vi "WPI_Camera Registry.vi"(8 "error in (no error)":errorcluster, 9 "Disallow Simulation":bool, 10 "Camera Address":string="192.168.0.90", 11 "Action":T2) -> (0 "error out":errorcluster, 3 "CameraDevRef":T1)   [LabVIEW 2017]
doc: "This software is licensed. Open the labview\\readme\\WPI Robotics Library Open Source License.txt file for more information."
uses:
  <vilib>/Rock Robotics/WPI/Camera/WPI_CameraRegistryActions.ctl
  <vilib>/Rock Robotics/WPI/Camera/WPI_CameraDevRef.ctl
  <vilib>/Rock Robotics/WPI/Camera/WPI_CameraSettings Operations.ctl
  <vilib>/Rock Robotics/WPI/Camera/WPI_CameraSettings Control.ctl
  <vilib>/Rock Robotics/WPI/Camera/WPI_CameraImageSize.ctl
  <vilib>/Rock Robotics/WPI/Camera/WPI_CameraWhite Balance Values.ctl
  <vilib>/Rock Robotics/WPI/Camera/WPI_CameraExposure Values.ctl
  <vilib>/Rock Robotics/WPI/Camera/WPI_CameraExposure Priority Values.ctl
  <vilib>/vision/driver/NI_Vision_Acquisition_Software.lvlib
panel:
  out "Camera Addresses":string[](array[string])
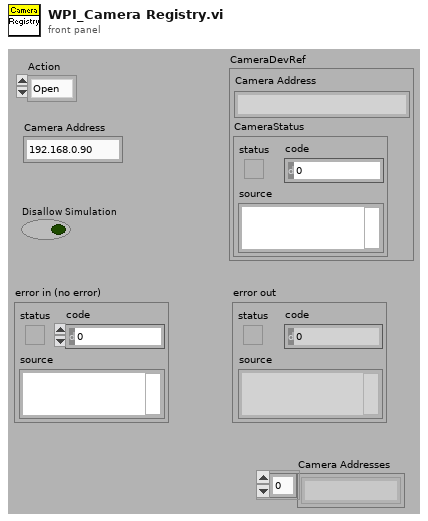
[diagram p1: front panel]
types:
  T1 = typedef "WPI_CameraDevRef.ctl" = cluster{"Camera Address":string, "CameraStatus":errorcluster}
  T2 = typedef "WPI_CameraRegistryActions.ctl" = enum16{"Open", "Close"}
  T3 = typedef "WPI_CameraSettings Control.ctl" = cluster{"FPS":i32, "Compression":i32, "Size":i32, "White Balance":i32, "Brightness":i32, "Sharpness":i32, "Exposure":i32, "Color Level":i32, "Exposure Priority":i32, "Color Enable":i32, "JPG Loop":i32, "MJPG Loop":i32, "Exposure Value":i32}
  T4 = typedef "WPI_CameraSettings Operations.ctl" = enum16{"Udate FPS", "Update Compression", "Update Size", "Update White Balance", "Update Brightness", "Update Sharpness", "Update Exposure", "Update Exposure Value", "Update Color Level", "Update Exp Priority", "Update Color Enable", "Update JPG", "Update MJPG", "Read and Clear", "Read", "Init"}
  T5 = typedef "WPI_CameraExposure Priority Values.ctl" = enum16{"None", "Prioritize frame rate", "Prioritize image quality"}
  T6 = typedef "WPI_CameraExposure Values.ctl" = enum16{"Auto", "Flicker-free 50 Hz", "Flicker-free 60 Hz", "Hold current", "Custom"}
  T7 = typedef "WPI_CameraWhite Balance Values.ctl" = enum16{"Auto", "Fixed indoor", "Fixed outdoor 1", "Fixed outdoor 2", "Fixed fluorescent 1", "Fixed fluorescent 2", "Hold current", "Custom"}
  T8 = typedef "WPI_CameraImageSize.ctl" = enum16{"640x480", "320x240", "160x120", "Custom"}
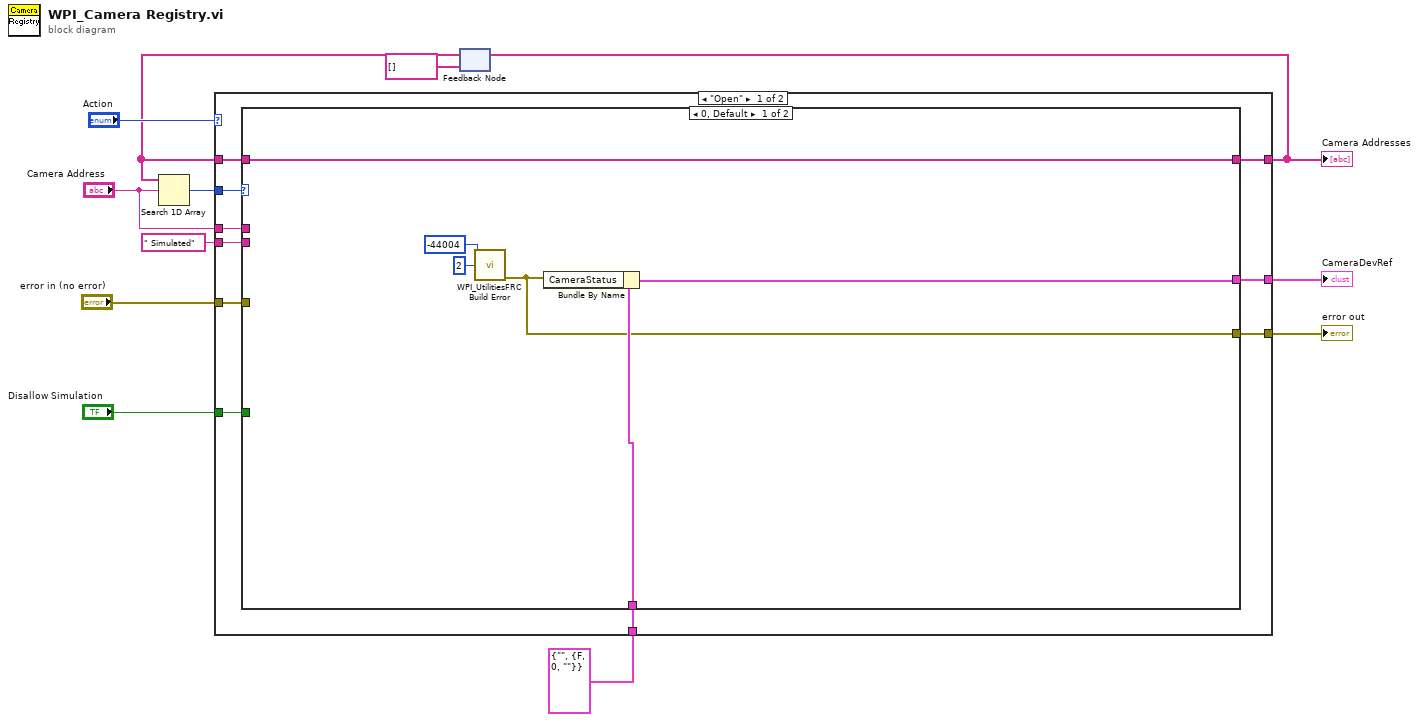
[diagram p0: block diagram]
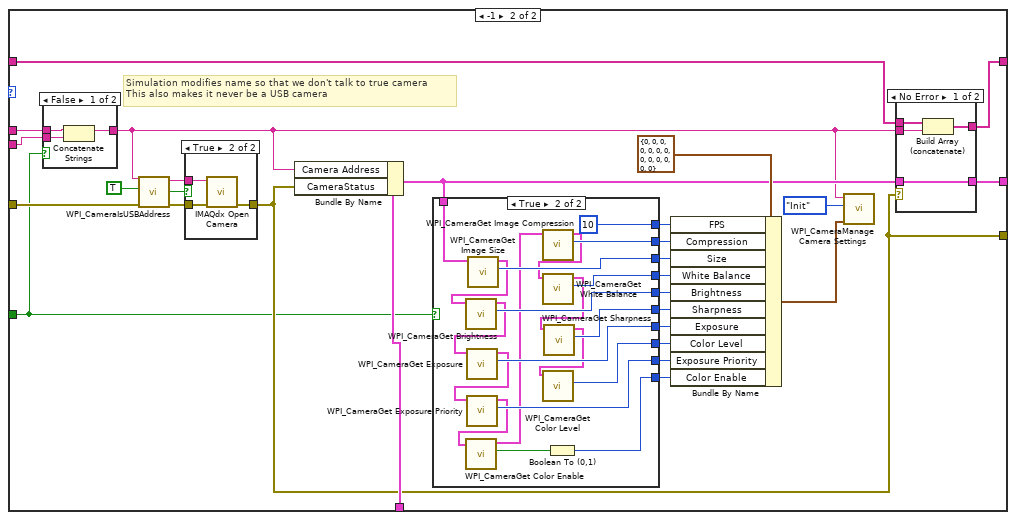
[diagram p2: hidden frame]
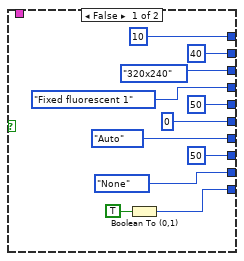
[diagram p4: hidden frame]
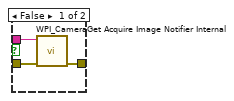
[diagram p5: hidden frame]
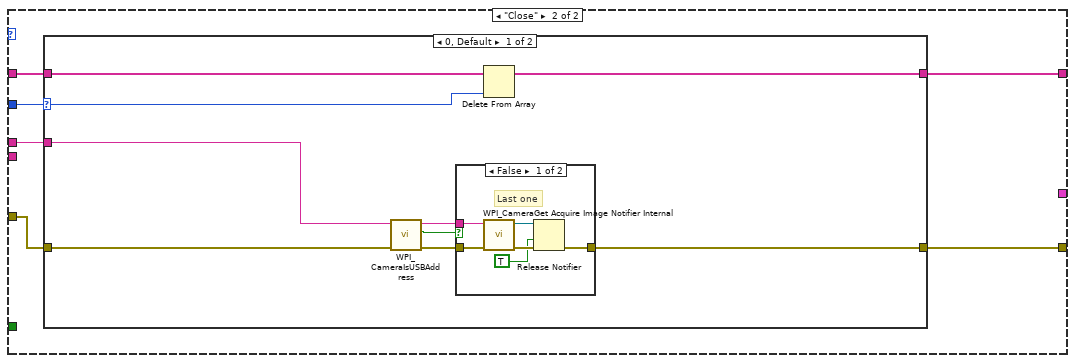
[diagram p7: hidden frame]
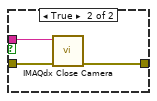
[diagram p8: hidden frame]
diagram:
  n1 = feedback #1(string[] []) -> (w6:string[])
  n2 = Search 1D Array(1D array=w6, element="Camera Address") -> (index of element=w7:i32)  [unwired: 1 out]
  n3 = case shown="\"Open\"" "Action" {
    tunnel: w6 -> [w21 w108]
    tunnel: "Camera Address" -> [w22 w105]
    tunnel: [w20 _] -> w11
    tunnel: w7 -> [w19 w109]
    tunnel: [w18 w107] -> w8
    tunnel: "error in (no error)" -> [w17 w104]
    tunnel: [w16 w106] -> w9
    tunnel: T1 {"Camera Address"="", "CameraStatus"={"status"=FALSE, "code"=0, "source"=""}} ("CameraDevRef") -> [w15 _]
    tunnel: "Disallow Simulation" -> [w14 _]
    tunnel: " Simulated" -> [w13 _]
    frame "Open" {
      n4 = case shown="0, Default" w19 {
        tunnel: w22 -> [_ w32]
        tunnel: w21 -> [w28 w56]
        tunnel: [w27 w54] -> w20
        tunnel: [w28 w55] -> w18
        tunnel: w17 -> [_ w36]
        tunnel: [w23 w51] -> w16
        tunnel: w15 -> [w26 w53]
        tunnel: w14 -> [_ w30]
        tunnel: w13 -> [_ w29]
        frame 0, Default {
          n5 = call <vilib>:"WPI_UtilitiesFRC Build Error.vi"("error code"=-44004 ("code"), "chain levels to remove (1)"=2) -> ("error out"=w23:errorcluster)  [unwired: 3 in, 10 out]
          n6 = Bundle By Name(cluster=w26, "CameraStatus"=w23) -> (w27:T1)
        }
        frame -1 {
          # "Simulation modifies name so that we don't talk to true camera\nThis also makes it never be a USB camera"
          n7 = case shown="False" w30 {
            tunnel: w32 -> [w59 w60]
            tunnel: [w57 w60] -> w31
            tunnel: w29 -> [w58 _]
            frame False {
              n8 = Concatenate Strings(w59, w58) -> (w57:string)
            }
            frame True {
            }
          }
          n9 = call <vilib>:"WPI_CameraIsUSBAddress.vi"("error in (no error)"=w36, "Enumerate?"=TRUE, "Camera Address In"=w31) -> ("error out"=w37:errorcluster, "USB?"=w34:bool, "Camera Address Out"=w35:string)  [unwired: 6 in]
          n10 = case shown="True" w34 {
            tunnel: w37 -> [w94 w97]
            tunnel: w35 -> [w93 w95]
            tunnel: [w92 w96] -> w51
            frame False {
              n11 = call <vilib>:"WPI_CameraGet Acquire Image Notifier Internal.vi"("error in (no error)"=w94, "Camera Address"=w93) -> ("error out"=w92:errorcluster)  [unwired: 9 out]
            }
            frame True {
              n12 = call <vilib>:"IMAQdx Open Camera.vi"("error in"=w97, "Session In"=w95) -> ("error out"=w96:errorcluster)  [unwired: 8 in, 1 out]
            }
          }
          n13 = Bundle By Name(cluster=w53, "Camera Address"=w31, "CameraStatus"=w51) -> (w38:T1)
          n14 = case shown="True" w30 {
            tunnel: [10 ("FPS") 10 ("FPS")] -> w50
            tunnel: [w70 w81] -> w47
            tunnel: [40 ("Compression") w88] -> w46
            tunnel: [WPI_CameraImageSize."320x240" ("Image Size") w89] -> w45
            tunnel: [WPI_CameraWhite_Balance_Values."Fixed fluorescent 1" ("White Balance") w87] -> w44
            tunnel: [50 ("Brightness") w86] -> w43
            tunnel: [0 ("Sharpness") w85] -> w42
            tunnel: [WPI_CameraExposure_Values."Auto" ("Exposure") w84] -> w41
            tunnel: [50 ("Color Level") w83] -> w40
            tunnel: [WPI_CameraExposure_Priority_Values."None" ("Exposure Priority") w82] -> w39
            tunnel: w38 -> [_ w76]
            frame False {
              n15 = Boolean To (0,1)(Boolean=TRUE ("Color Enabled")) -> (0, 1=w70:i16)
            }
            frame True {
              n16 = call <vilib>:"WPI_CameraGet Image Size.vi"("CameraDevRef"=w76) -> ("Image Size"=w89:T8, "CameraDevRef Out"=w80:T1)  [unwired: 7 in, 2 out]
              n17 = call <vilib>:"WPI_CameraGet Brightness.vi"("CameraDevRef"=w80) -> ("Brightness"=w86:i32, "CameraDevRef Out"=w79:T1)  [unwired: 8 in, 1 out]
              n18 = call <vilib>:"WPI_CameraGet Exposure.vi"("CameraDevRef"=w79) -> ("Exposure"=w84:T6, "CameraDevRef Out"=w78:T1)  [unwired: 7 in, 2 out]
              n19 = call <vilib>:"WPI_CameraGet Exposure Priority.vi"("CameraDevRef"=w78) -> ("Exposure Priority"=w82:T5, "CameraDevRef Out"=w77:T1)  [unwired: 8 in, 1 out]
              n20 = call <vilib>:"WPI_CameraGet Color Enable.vi"("CameraDevRef"=w77) -> ("Color Enabled"=w91:bool, "CameraDevRef Out"=w75:T1)  [unwired: 8 in, 1 out]
              n21 = call <vilib>:"WPI_CameraGet Image Compression.vi"("CameraDevRef"=w75) -> ("Compression"=w88:i32, "CameraDevRef Out"=w74:T1)  [unwired: 8 in, 1 out]
              n22 = call <vilib>:"WPI_CameraGet White Balance.vi"("CameraDevRef"=w74) -> ("White Balance"=w87:T7, "CameraDevRef Out"=w73:T1)  [unwired: 7 in, 2 out]
              n23 = call <vilib>:"WPI_CameraGet Sharpness.vi"("CameraDevRef"=w73) -> ("Sharpness"=w85:i32, "CameraDevRef Out"=w72:T1)  [unwired: 8 in, 1 out]
              n24 = call <vilib>:"WPI_CameraGet Color Level.vi"("CameraDevRef"=w72) -> ("Color Level"=w83:i32)  [unwired: 8 in, 2 out]
              n25 = Boolean To (0,1)(Boolean=w91) -> (0, 1=w81:i16)
            }
          }
          n26 = Bundle By Name(cluster=T3 {"FPS"=0, "Compression"=0, "Size"=0, "White Balance"=0, "Brightness"=0, "Sharpness"=0, "Exposure"=0, "Color Level"=0, "Exposure Priority"=0, "Color Enable"=0, "JPG Loop"=0, "MJPG Loop"=0, "Exposure Value"=0} ("Values In"), "FPS"=w50, "Compression"=w46, "Size"=w45, "White Balance"=w44, "Brightness"=w43, "Sharpness"=w42, "Exposure"=w41, "Color Level"=w40, "Exposure Priority"=w39, "Color Enable"=w47) -> (w48:T3)
          n27 = call <vilib>:"WPI_CameraManage Camera Settings.vi"("Values In"=w48, "Operation"=WPI_CameraSettings_Operations."Init", "Camera IP"=w31) -> ()  [unwired: 7 in, 2 out]
          n28 = case shown="No Error" w51 {
            tunnel: w56 -> [w101 w103]
            tunnel: w31 -> [w100 _]
            tunnel: w38 -> [w98 w102]
            tunnel: [w99 w103] -> w55
            tunnel: [w98 w102] -> w54
            frame No Error {
              n29 = Build Array (concatenate)(w101, w100) -> (w99:string[])
            }
            frame Error {
            }
          }
        }
      }
    }
    frame "Close" {
      n30 = case shown="0, Default" w109 {
        selector: w109 -> [w115 _]
        tunnel: w108 -> [w118 w129]
        tunnel: [w117 w129] -> w107
        tunnel: w104 -> [w110 w128]
        tunnel: [w116 w128] -> w106
        tunnel: w105 -> [w111 _]
        frame 0, Default {
          n31 = call <vilib>:"WPI_CameraIsUSBAddress.vi"("error in (no error)"=w110, "Camera Address In"=w111) -> ("error out"=w113:errorcluster, "USB?"=w114:bool, "Camera Address Out"=w112:string)  [unwired: 7 in]
          n32 = case shown="False" w114 {
            tunnel: w113 -> [w124 w126]
            tunnel: [w123 w125] -> w116
            tunnel: w112 -> [w119 w127]
            frame False {
              # "Last one"
              n33 = call <vilib>:"WPI_CameraGet Acquire Image Notifier Internal.vi"("error in (no error)"=w124, "Camera Address"=w119) -> ("error out"=w122:errorcluster, "Acquire Image Notifier"=w121:refnum<notifier>)  [unwired: 8 out]
              n34 = Release Notifier(notifier=w121, force destroy? (F)=TRUE, error in (no error)=w122) -> (error out=w123:errorcluster)  [unwired: 2 out]
            }
            frame True {
              n35 = call <vilib>:"IMAQdx Close Camera.vi"("error in"=w126, "Session In"=w127) -> ("error out"=w125:errorcluster)  [unwired: 9 in]
            }
          }
          n36 = Delete From Array(array=w118, index=w115) -> (array with subset deleted=w117:string[])  [unwired: 1 in, 1 out]
        }
        frame -1 {
        }
      }
    }
  }
  "CameraDevRef" <- w11
  "error out" <- w9
  "Camera Addresses" <- w8
  n37 = feedback-in #1(w8) -> ()
